vi "Set Variables.vi"(8 "error in (no error)":errorcluster, 10 "Variables":variant, 11 "Comparison Popup in":refnum<class "Comparison Functions.lvclass">) -> (0 "error out":errorcluster, 3 "Comparison Popup out":refnum<class "Comparison Functions.lvclass">)   [LabVIEW 2016, in "Comparison Functions.lvclass"]
uses:
  Comparison Functions.lvclass
  Comparison Functions.lvclass/Comparison Functions.ctl
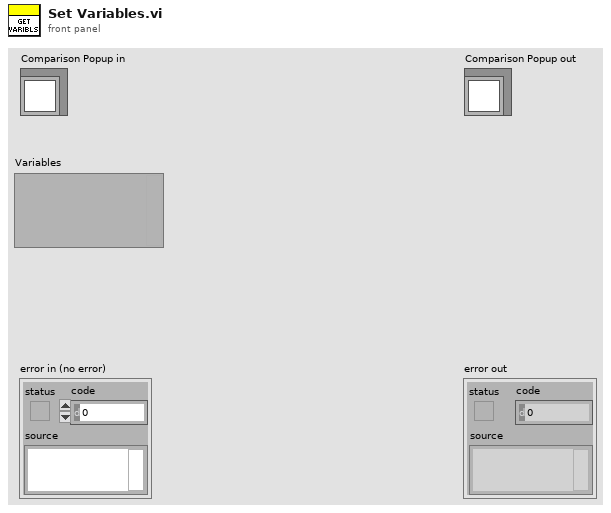
[diagram p1: front panel]
types:
  T1 = typedef "Comparison Functions.lvclass/Variables.ctl" = cluster{"Var1":variant, "Var2":variant}
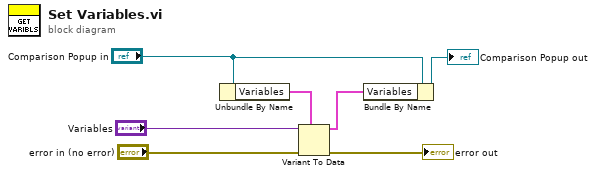
[diagram p0: block diagram]
diagram:
  n1 = Unbundle By Name("Comparison Popup in") -> ("Variables"=w2:T1)
  n2 = Variant To Data(error in="error in (no error)", type=w2, Variant="Variables") -> (data=w1:T1, error out=→"error out":errorcluster)
  n3 = Bundle By Name(cluster="Comparison Popup in", "Variables"=w1) -> (→"Comparison Popup out":refnum<class "Comparison Functions.lvclass">)
